vi "tearDown.vi"(8 "error in (no error)":errorcluster, 11 "reference in":refnum<class "SLSC Switch Export Unit Tests.lvclass">) -> (0 "error out":errorcluster, 3 "reference out":refnum<class "SLSC Switch Export Unit Tests.lvclass">)   [LabVIEW 2017, in "SLSC Switch Export Unit Tests.lvclass"]
doc: "tearDown runs after the test method has completed. Use this method to clean up any operations or references that were opened by setUp or the test method. Unit tests should be independent of other unit tests so this VI should ensure that the next test can run in a 'clean' test environment."
uses:
  SLSC Switch Export Unit Tests.lvclass
  SLSC Switch Export Unit Tests.lvclass/SLSC Switch Export Unit Tests.ctl
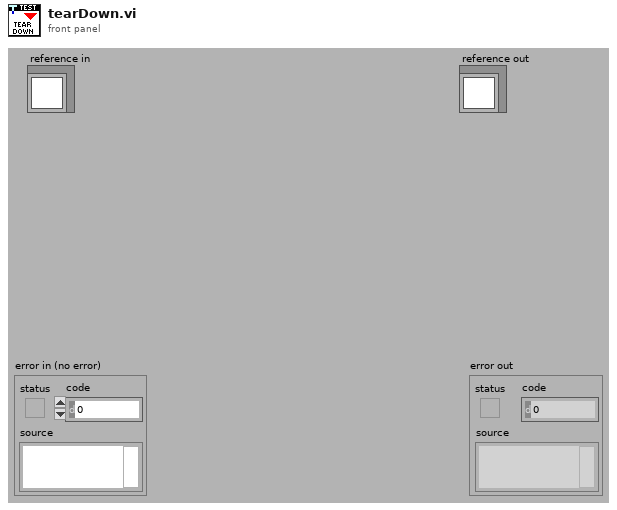
[diagram p1: front panel]
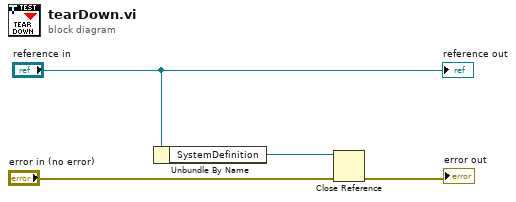
[diagram p0: block diagram]
diagram:
  n1 = Unbundle By Name("reference in") -> ("SystemDefinition"=w2:refnum<k24>)
  n2 = Close Reference(reference=w2, error in (no error)="error in (no error)") -> (error out=→"error out":errorcluster)
  "reference out" <- "reference in"
